vi "Get Background Colors - constant.vi"() -> (0 "Color":u32(colorbox))   [LabVIEW 2020, in "Run Utilities.lvlib" / "Schedule Block.lvclass"]
doc: "Each time this VI is run, it returns next out of list of 5 colors. This is used for setting background color of the GUI elements"
uses:
  Schedule Block.lvclass
  Schedule Block.lvclass/Schedule Block.ctl
panel:
  in  "index":i32
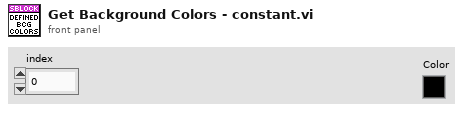
[diagram p1: front panel]
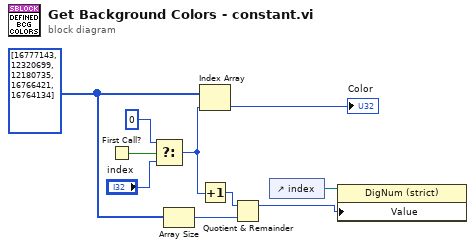
[diagram p0: block diagram]
diagram:
  w10 = u32[] [16777143, 12320699, 12180735, 16766421, 16764134] ("Colors")
  n1 = First Call?() -> (First Call?: T/F=w2:bool)
  n2 = Select(t=0, s=w2, f="index") -> (s? t:f=w4:i32)
  n3 = Array Size(array=w10) -> (size(s)=w9:i32)
  n4 = Index Array(array=w10, index=w4) -> (element=→"Color":u32)
  n5 = Increment(x=w4) -> (x+1=w5:i32)
  n6 = Quotient & Remainder(x=w5, y=w9) -> (x-y*floor(x/y)=w7:i32)  [unwired: 1 out]
  n7 = control-ref of="index"() -> (w8:refnum<vi>)
  n8 = property class="DigNum (strict)"(reference=w8, "Value"=w7) -> ()  [unwired: 1 in, 2 out]
